vi "SubPanel VI external control thread.vi"(8 "error in (no error)":errorcluster, 9 "index":i32=3, 11 "Control Data":T1={"Queue Array"=[], "Queue Element"={"state"="", "data"=variant}, "System Event"=refnum, "System Event RefNum"=refnum, "Queue List"=[], "LPCA COM"="", "Rotating"=FALSE, "PrecorAI"="", "T_0 Index"=0, "Bar Graph X"=[], "Channels"=[], "Active Indicies"=[], "Active Channels"=[], "Sample Frequency"=0.0, "Ibrake Sweep"=[], "RPM Sweep"=[], "Load Sweep"=[], "Step Height Sweep"=[], "Range Sweep"=[], "A Counter"=0, "B Counter"=0, "C Counter"=0, "#A"=0, "#B"=0, "#C"=0, "Current RPM"=0.0, "Current Ibrake"=0, "Current Range"=0, "Current Step Height"=0, "Load Bank"=enum."OFF", "Cfg Cntrls"=[], "T_Monitor Indices"=[], "Thermal Limit"=0, "Thermal Resume"=0, "Timer Reset"=FALSE, "Stop Time"=0.0, "Autotest"=FALSE, "Pulsed RPM Capture"=FALSE, "Get Sample"=FALSE, "Last State"="", "Reset Timeout"=FALSE, "Ctrl Refs"={"Test Details"=refnum, "Save Config"=refnum, "Load Config"=refnum, "Path"=refnum, "Snapshot"=refnum, "SS#"=refnum, "Ibrake"=refnum, "RPM Target"=refnum, "Spin"=refnum, "Load Bank"=refnum, "Start Test"=refnum, "Pause Test"=refnum, "Load Sweep"=refnum, "RPM Sweep"=refnum, "Ibrake Sweep"=refnum, "Filters"=refnum, "Sample Frequency"=refnum, "Data Setup"=refnum, "Pause"=refnum, "Stop Time"=refnum, "S Period"=refnum, "Range"=refnum, "Step Height"=refnum, "Step Height Sweep"=refnum, "Range Sweep"=refnum, "Available Tests"=refnum, "RPM Graph"=refnum, "RPM Knob"=refnum, "FanMode"=refnum, "Fan Mode LED Array"=refnum, "Thermal Equilibrium"=refnum, "Data Display"=refnum, "LPCA Error"=refnum, "LPCA Ramp"=refnum, "LPCA Range"=refnum, "LPCA Resistance"=refnum, "Analyze Read"=refnum, "Console Select"=refnum, "Sub Panel"=refnum}, "Pulse Waveform"={"t0"=timestamp(0 s since 1904-01-01), "dt"=1.0, "Y"=[]}, "Snapshot"={"Test Details"="test", "Version"="test", "Date"=timestamp(3493915594.3018084 s since 1904-01-01), "Selected Test"="man", "Snapshot Number"=0, "Time"=timestamp(3493915602.7292905 s since 1904-01-01), "Ibrake Setpoint"="1", "RPM Setpoint"="20", "Range Setpoint"="", "Step Height Setpoint"="", "Load Bank Setpoint"="15", "Measurement Headers"="a,b,c,1,2,3", "Measurements"="1,2,3,4,5,6,7,8", "A"=0, "B"=0, "C"=0, "Raw Data"=[], "Available Tests"=enum."Manual", "Ibrake List"="", "RPM List"="", "Load Bank List"="", "Range List"="", "Step Height List"="", "FanMode Setpoint"=enum."Auto"}, "Sample Period"=0.0, "OverTemp"=FALSE, "Available Tests"=enum."Manual", "FanMode"=enum."Auto", "Fan Mode LED Array"=[FALSE, TRUE, FALSE], "Thermal\nEquilibrium "=FALSE, "Equilibrium Stop"=FALSE, "AvgDegChg"=[]} {"Snapshot"."Time" format="%<%H:%M:%S>T"; "Snapshot"."Date" format="%<%m/%d/%Y>T"}) -> ()   [LabVIEW 2017]
uses:
  Source/Controls/Test TypeDef.ctl
  Queue References Array.ctl
  Queue Element.ctl
  Source/Controls/Load Bank.ctl
  Source/Controls/Available Tests.ctl
  Source/Console Sim/Controls/Console Select.ctl
  Source/Controls/Snapshot Typedef.ctl
  Source/Controls/FanMode.ctl
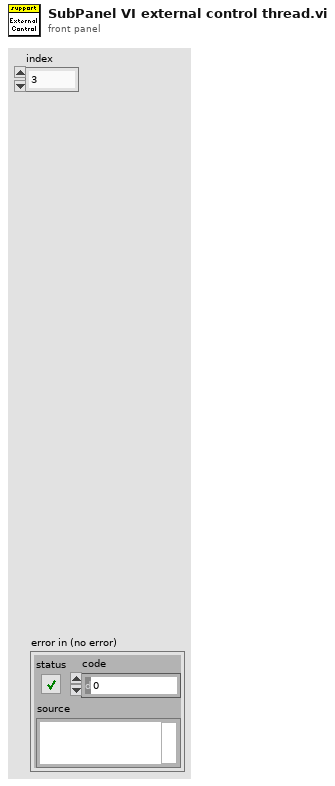
[diagram p1: front panel]
types:
  T1 = typedef "Test TypeDef.ctl" = cluster{"Queue Array":T2, "Queue Element":T3, "System Event":refnum<user-event>, "System Event RefNum":refnum<event-registration>, "Queue List":string[], "LPCA COM":refnum<visa-resource-name>, "Rotating":bool, "PrecorAI":refnum<k21>, "T_0 Index":i32, "Bar Graph X":i32[], "Channels":string[], "Active Indicies":i32[], "Active Channels":string[][], "Sample Frequency":dbl, "Ibrake Sweep":string[], "RPM Sweep":string[], "Load Sweep":string[], "Step Height Sweep":string[], "Range Sweep":string[], "A Counter":i32, "B Counter":i32, "C Counter":i32, "#A":i32, "#B":i32, "#C":i32, "Current RPM":dbl, "Current Ibrake":u32, "Current Range":u32, "Current Step Height":u32, "Load Bank":T4, "Cfg Cntrls":refnum<vi>[], "T_Monitor Indices":i32[], "Thermal Limit":i32, "Thermal Resume":i32, "Timer Reset":bool, "Stop Time":dbl, "Autotest":bool, "Pulsed RPM Capture":bool, "Get Sample":bool, "Last State":string, "Reset Timeout":bool, "Ctrl Refs":cluster{"Test Details":refnum<vi>, "Save Config":refnum<vi>, "Load Config":refnum<vi>, "Path":refnum<vi>, "Snapshot":refnum<vi>, "SS#":refnum<vi>, "Ibrake":refnum<vi>, "RPM Target":refnum<vi>, "Spin":refnum<vi>, "Load Bank":refnum<vi>, "Start Test":refnum<vi>, "Pause Test":refnum<vi>, "Load Sweep":refnum<vi>, "RPM Sweep":refnum<vi>, "Ibrake Sweep":refnum<vi>, "Filters":refnum<vi>, "Sample Frequency":refnum<vi>, "Data Setup":refnum<vi>, "Pause":refnum<vi>, "Stop Time":refnum<vi>, "S Period":refnum<vi>, "Range":refnum<vi>, "Step Height":refnum<vi>, "Step Height Sweep":refnum<vi>, "Range Sweep":refnum<vi>, "Available Tests":refnum<vi>, "RPM Graph":refnum<vi>, "RPM Knob":refnum<vi>, "FanMode":refnum<vi>, "Fan Mode LED Array":refnum<vi>, "Thermal Equilibrium":refnum<vi>, "Data Display":refnum<vi>, "LPCA Error":refnum<vi>, "LPCA Ramp":refnum<vi>, "LPCA Range":refnum<vi>, "LPCA Resistance":refnum<vi>, "Analyze Read":refnum<vi>, "Console Select":refnum<vi>, "Sub Panel":refnum<vi>}, "Pulse Waveform":waveform(dbl), "Snapshot":T5, "Sample Period":dbl, "OverTemp":bool, "Available Tests":T6, "FanMode":T7, "Fan Mode LED Array":bool[], "Thermal\nEquilibrium ":bool, "Equilibrium Stop":bool, "AvgDegChg":dbl[]}
  T2 = typedef "Queue References Array.ctl" = refnum<queue>[]
  T3 = typedef "Queue Element.ctl" = cluster{"state":string, "data":variant}
  T4 = typedef "Load Bank.ctl" = enum16{"OFF", "50", "25", "16.7", "12.5", "10.0", "8.3", "7.1", "6.3", "5.6", "5.0", "4.5", "4.2", "3.8", "3.6", "3.3", "3.1"}
  T5 = typedef "Snapshot Typedef.ctl" = cluster{"Test Details":string, "Version":string, "Date":timestamp, "Selected Test":string, "Snapshot Number":u16, "Time":timestamp, "Ibrake Setpoint":string, "RPM Setpoint":string, "Range Setpoint":string, "Step Height Setpoint":string, "Load Bank Setpoint":string, "Measurement Headers":string, "Measurements":string, "A":i32, "B":i32, "C":i32, "Raw Data":string[][], "Available Tests":T6, "Ibrake List":string, "RPM List":string, "Load Bank List":string, "Range List":string, "Step Height List":string, "FanMode Setpoint":T7}
  T6 = typedef "Available Tests.ctl" = enum16{"Manual", "EFX Brake Torque", "Generator Torque", "EFX Brake Thermal", "Generator Thermal", "Pulsed RPM", "AMT Brake Torque", "Bike Brake Torque", "AMT Brake Thermal", "Bike Brake Thermal"}
  T7 = typedef "FanMode.ctl" = enum16{"On", "Off", "Auto"}
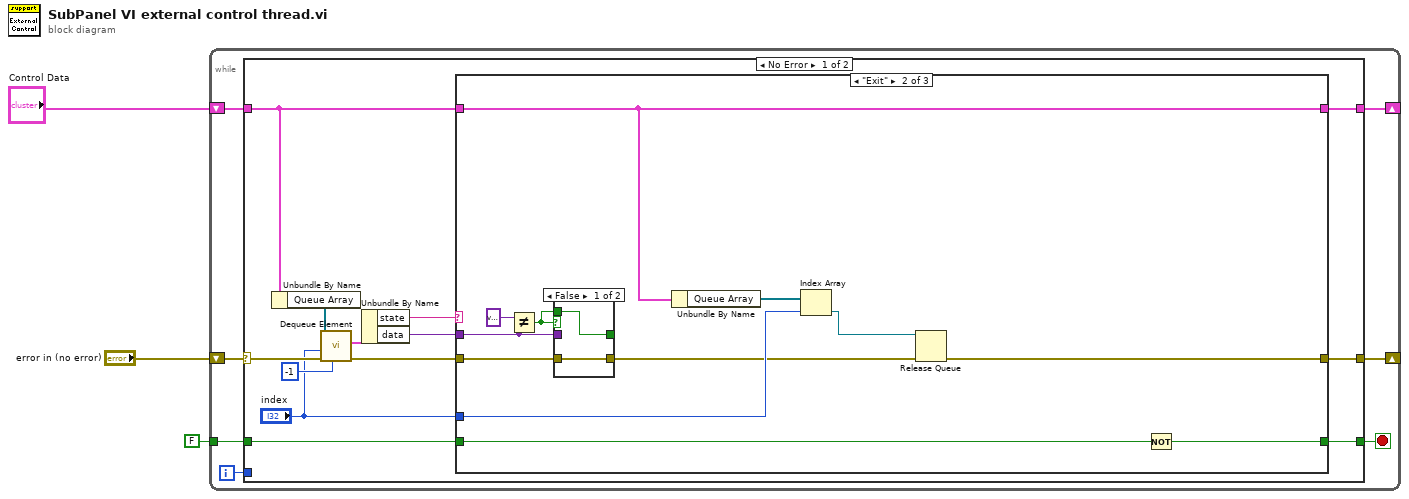
[diagram p0: block diagram]
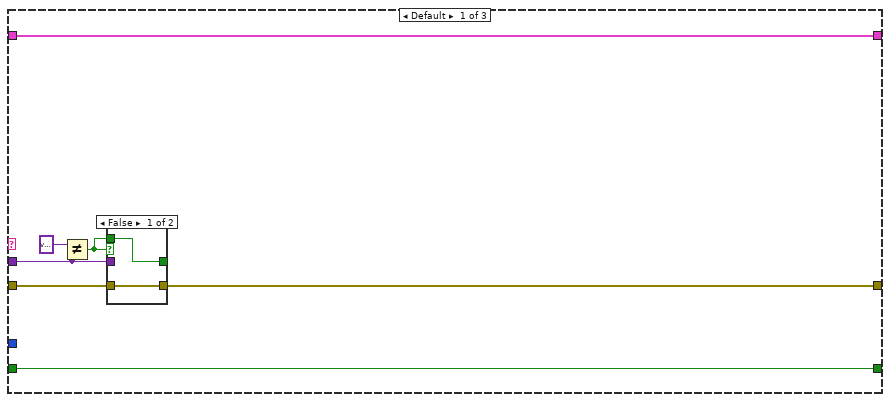
[diagram p2: hidden frame]
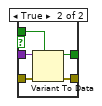
[diagram p3: hidden frame]
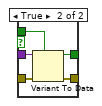
[diagram p4: hidden frame]
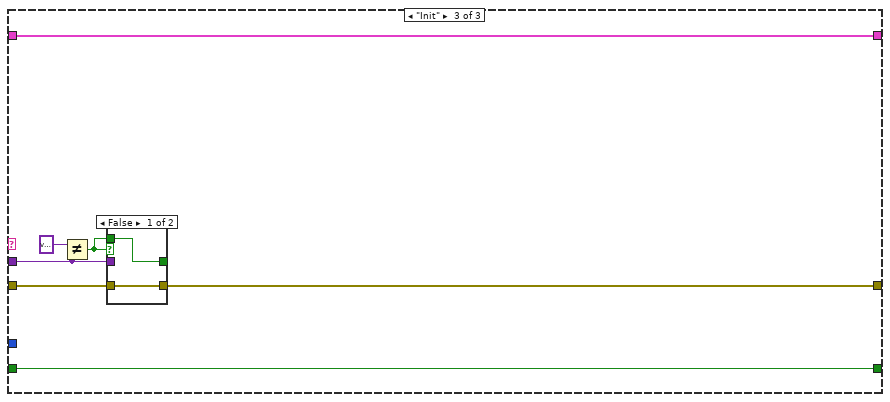
[diagram p5: hidden frame]
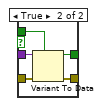
[diagram p6: hidden frame]
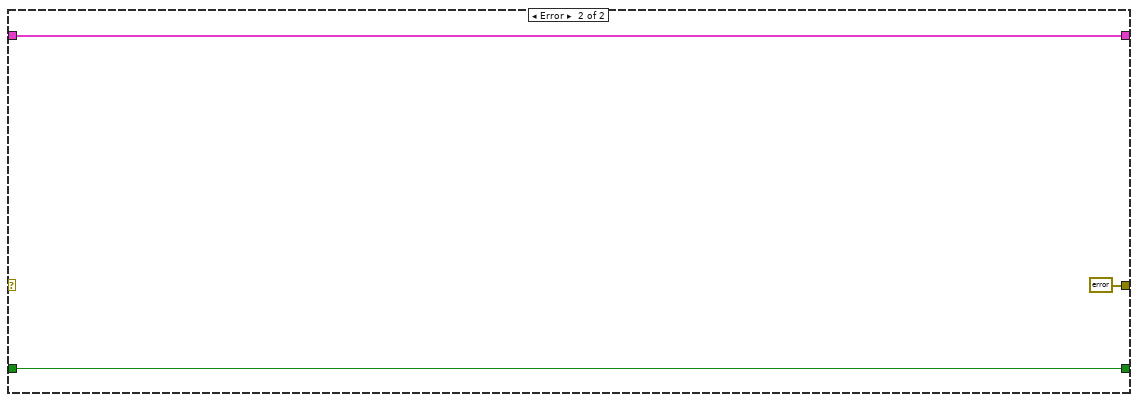
[diagram p7: hidden frame]
diagram:
  n1 = while {
    shift-right: [w5] -> _
    shift-left: "Control Data" -> [w10]
    tunnel: FALSE ("Boolean") -> [w7]
    shift-right: [w8] -> _
    shift-left: "error in (no error)" -> [w9]
    i -> [w4]
    stop <- w6 stop-if-true
    n2 = case shown="No Error" w9 {
      selector: w9 -> [w21 _]
      tunnel: w10 -> [w13 w73]
      tunnel: [w19 errorcluster {"status"=FALSE, "code"=0, "source"=""} ("error out")] -> w8
      tunnel: w7 -> [w18 w72]
      tunnel: [w17 w72] -> w6
      tunnel: [w14 w73] -> w5
      tunnel: w4 -> [_ _]
      frame No Error {
        n3 = Unbundle By Name(w13) -> ("Queue Array"=w23:T2)
        n4 = call "Dequeue Element.vi"("timeout in ms (-1)"=-1, "error in (no error)"=w21, "index"="index", "Queue Array"=w23) -> ("error out"=w20:errorcluster, "Queue Element"=w12:T3)  [unwired: 5 in, 1 out]
        n5 = Unbundle By Name(w12) -> ("state"=w16:string, "data"=w15:variant)
        n6 = case shown="\"Exit\"" w16 {
          tunnel: w20 -> [w28 w48 w62]
          tunnel: [w27 w38 w57] -> w19
          tunnel: w18 -> [w30 w49 w63]
          tunnel: [w30 w44 w63] -> w17
          tunnel: w15 -> [w25 w46 w60]
          tunnel: [w29 w43 w58] -> w14
          tunnel: w13 -> [w29 w43 w58]
          tunnel: "index" -> [_ w41 _]
          frame Default {
            n7 = Not Equal?(x=variant, y=w25) -> (x != y?=w24:bool)
            n8 = case shown="False" w24 {
              tunnel: w28 -> [w32 w37]
              tunnel: [w32 w36] -> w27
              tunnel: w25 -> [_ w35]
              tunnel: [w31 w34] -> _
              tunnel: w24 -> [w31 w33]
              frame False {
              }
              frame True {
                n9 = Variant To Data(error in=w37, type=w33, Variant=w35) -> (data=w34:bool, error out=w36:errorcluster)
              }
            }
          }
          frame "Exit" {
            n10 = Not Equal?(x=variant, y=w46) -> (x != y?=w45:bool)
            n11 = case shown="False" w45 {
              tunnel: w48 -> [w51 w56]
              tunnel: [w51 w55] -> w39
              tunnel: w46 -> [_ w54]
              tunnel: [w50 w53] -> _
              tunnel: w45 -> [w50 w52]
              frame False {
              }
              frame True {
                n12 = Variant To Data(error in=w56, type=w52, Variant=w54) -> (data=w53:bool, error out=w55:errorcluster)
              }
            }
            n13 = Unbundle By Name(w43) -> ("Queue Array"=w42:T2)
            n14 = Index Array(array=w42, index=w41) -> (element=w40:refnum<queue>)
            n15 = Release Queue(queue=w40, error in (no error)=w39) -> (error out=w38:errorcluster)  [unwired: 1 in, 2 out]
            n16 = Not(x=w49) -> (.not. x?=w44:bool)
          }
          frame "Init" {
            n17 = Not Equal?(x=variant, y=w60) -> (x != y?=w59:bool)
            n18 = case shown="False" w59 {
              tunnel: w62 -> [w65 w70]
              tunnel: [w65 w69] -> w57
              tunnel: w60 -> [_ w68]
              tunnel: [w64 w67] -> _
              tunnel: w59 -> [w64 w66]
              frame False {
              }
              frame True {
                n19 = Variant To Data(error in=w70, type=w66, Variant=w68) -> (data=w67:bool, error out=w69:errorcluster)
              }
            }
          }
        }
      }
      frame Error {
      }
    }
  }
